vi "Get GUID.vi"(8 "error in (no error)":errorcluster, 11 "Hardware in":refnum<class "Hardware.lvclass">) -> (0 "error out":errorcluster, 2 "GUID":string, 3 "Hardware out":refnum<class "Hardware.lvclass">)   [LabVIEW 2016, in "Hardware.lvlib" / "Hardware.lvclass"]
uses:
  <userlib>/Common Components/Hardware/Abstract Hardware/Hardware.lvclass
  <userlib>/Common Components/Hardware/Abstract Hardware/Hardware.lvclass/Hardware.ctl
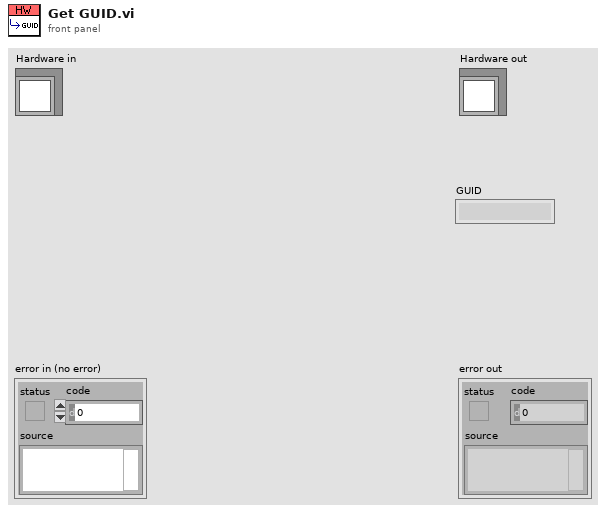
[diagram p1: front panel]
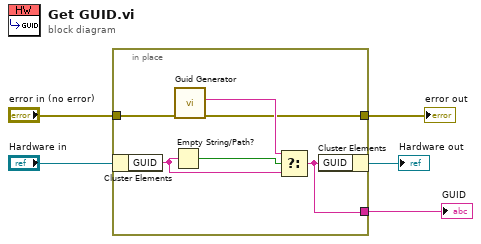
[diagram p0: block diagram]
diagram:
  n1 = in-place {
    in-place-border: "error in (no error)" -> [w8]
    in-place-border: [w7] -> w2
    in-place-border: [w6] -> w1
    n2 = in-place-cluster #1("Hardware in") -> ("GUID"=w9:string)
    n3 = Empty String/Path?(string/path=w9) -> (empty?=w11:bool)
    n4 = call <vilib>:"Guid Generator.vi"("error in (no error)"=w8) -> ("error out"=w7:errorcluster, "GUID"=w10:string)  [unwired: 9 in]
    n5 = Select(t=w10, s=w11, f=w9) -> (s? t:f=w6:string)
    n6 = in-place-cluster #1("GUID"=w6) -> (→"Hardware out":refnum<class "Hardware.lvclass">)
  }
  "error out" <- w2
  "GUID" <- w1
